vi "genererfrekvenssignal0.2.vi"() -> ()   [LabVIEW 2014]
panel:
  out "The given frequency:":dbl(slide) scale=800.0..2000.0
  in  "Enter frequency:":dbl
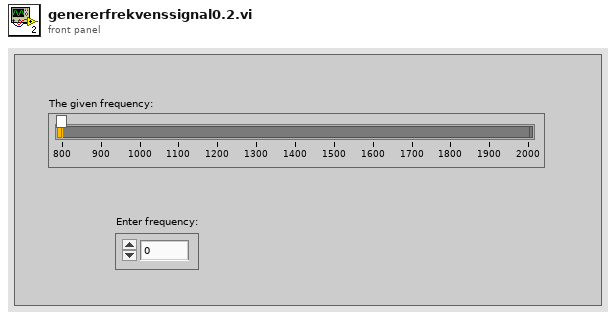
[diagram p1: front panel]
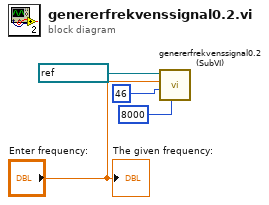
[diagram p0: block diagram]
diagram:
  n1 = call "genererfrekvenssignal0.2(SubVI).vi"("Duration (ms)"=u32 8000, "Channel"=u8 46, "Enter frequency:"="Enter frequency:", "VISA Refnum in"=refnum<visa-resource-name> "Højtaler" ("Serial Port")) -> ()  [unwired: 8 in]
  "The given frequency:" <- "Enter frequency:"
